vi "UDP SENDER.vi"(6 "queue":refnum<queue>, 7 "milliseconds to wait (LoopTimer)":u32, 8 "error in (no error)":errorcluster, 9 "destination adress":string, 10 "destination port":u16, 11 "UDP Network Connection in":refnum<k16>) -> (0 "error out":errorcluster)   [LabVIEW 2016]
uses:
  Globale Variablen VI/AutonomousMode.vi
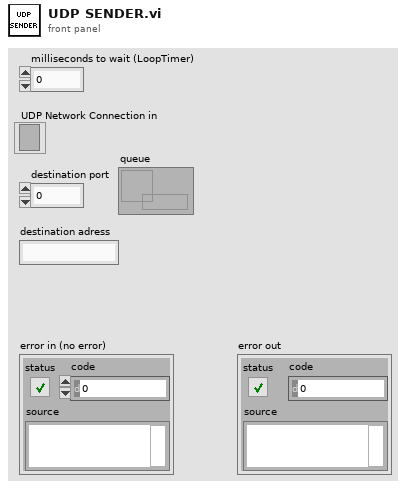
[diagram p1: front panel]
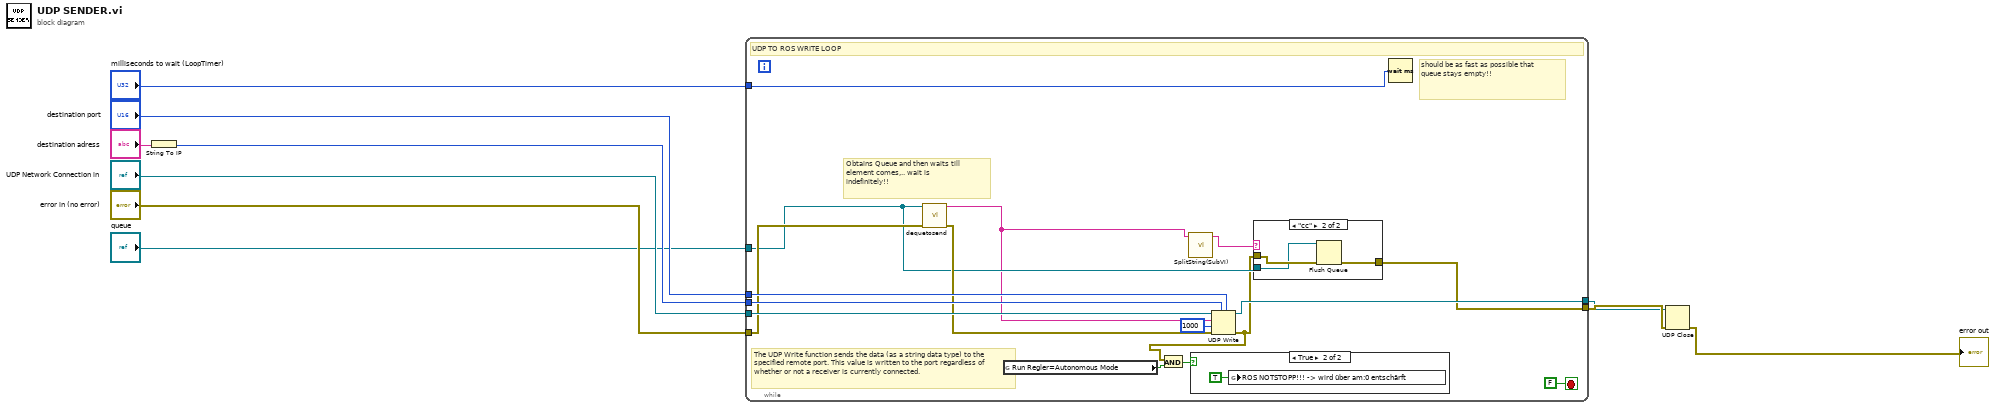
[diagram p0: block diagram]
diagram:
  n1 = String To IP(1:"destination adress") -> (0:w7:u32)
  n2 = while {
    tunnel: [w17] -> w9
    tunnel: "destination port" -> [w26]
    tunnel: w7 -> [w25]
    tunnel: "UDP Network Connection in" -> [w24]
    tunnel: "error in (no error)" -> [w21]
    tunnel: [w23] -> w8
    tunnel: "milliseconds to wait (LoopTimer)" -> [w22]
    tunnel: "queue" -> [w18]
    stop <- FALSE stop-if-true
    # "should be as fast as possible that queue stays empty!!"
    # "Obtains Queue and then waits till element comes,.. wait is indefinitely!!"
    # "The UDP Write function sends the data (as a string data type) to the specified remote port. This value is written to the port regardless of whether or not a receiver is currently connected."
    # "UDP TO ROS WRITE LOOP"
    n3 = call "dequetosend.vi"("error in (no error)"=w21, "queue"=w18) -> ("error out"=w20:errorcluster, "String to be sent"=w16:string)  [unwired: 8 in]
    n4 = global read "AutonomousMode.vi" "Run Regler=Autonomous Mode"() -> (w13:bool)
    n5 = call "SplitString(SubVI).vi"("data in"=w16) -> ("String 3"=w15:string)  [unwired: 9 in, 1 out]
    n6 = UDP Write(address=w25, port or service name=w26, connection ID=w24, data in=w16, 8:w20, 9:1000 ("timeout ms (25000)")) -> (error out=w12:errorcluster, 3:w23:refnum<k16>)
    n7 = And(x=w12, y=w13) -> (x .and. y?=w14:bool)
    n8 = case shown="True" w14 {
      frame False {
      }
      frame True {
        n9 = global write "AutonomousMode.vi" "ROS NOTSTOPP!!! -> wird über am:0 entschärft"(TRUE ("ROS NOTSTOPP!!! -> wird über am:0 entschärft")) -> ()
      }
    }
    n10 = case shown="\"cc\"" w15 {
      tunnel: w18 -> [_ w30]
      tunnel: w12 -> [w28 w31]
      tunnel: [w28 w29] -> w17
      frame Default {
      }
      frame "cc" {
        n11 = Flush Queue(queue=w30, error in (no error)=w31) -> (error out=w29:errorcluster)  [unwired: 2 out]
      }
    }
    n12 = Wait (ms)(milliseconds to wait=w22) -> ()  [unwired: 1 out]
  }
  n13 = UDP Close(connection ID=w8, 8:w9) -> (error out=→"error out":errorcluster)  [unwired: 1 out]
